vi "LVClass_WavefrontCorrector Reset to Factory WavefrontCorrectorSet.vi"(0 "WavefrontCorrector in":refnum<class "WavefrontCorrector.lvclass">, 5 "load_and_apply_connection_params":bool, 7 "load_and_apply_params":bool, 11 "error in (no error)":errorcluster) -> (4 "WavefrontCorrector out":refnum<class "WavefrontCorrector.lvclass">, 15 "error out":errorcluster)   [LabVIEW 2020, in "WavefrontCorrector.lvclass"]
doc: "Wavefront corrector parameter getter for parameter of type string.\n\n--------------------------------------------------------------------------------\n\n<B>correctorIn </B> : WavefrontCorrector object.\n<B>correctorOut </B> : WavefrontCorrector object.\n<B>parameter_name </B> : Name of the parameter.\n<B>value </B> : Value of the parameter.\n<B>ErrorIn </B> : Error\n<B>ErrorOut </B> : Error\n\n--------------------------------------------------------------------------------"
uses:
  WavefrontCorrector.lvclass
  WavefrontCorrector.lvclass/WavefrontCorrector.ctl
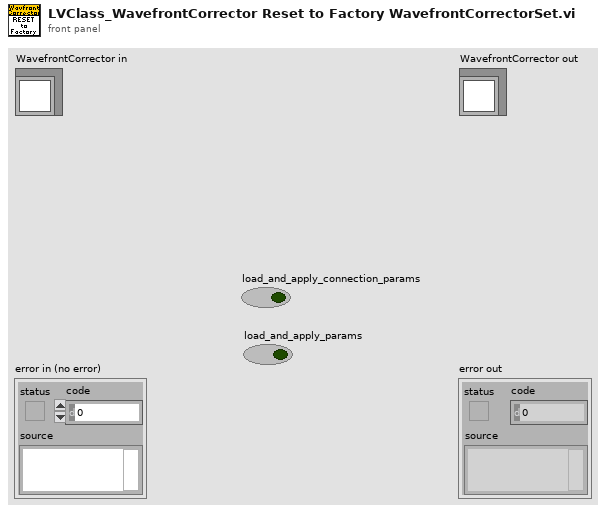
[diagram p1: front panel]
types:
  T1 = typedef "ClassID.ctl" = i64
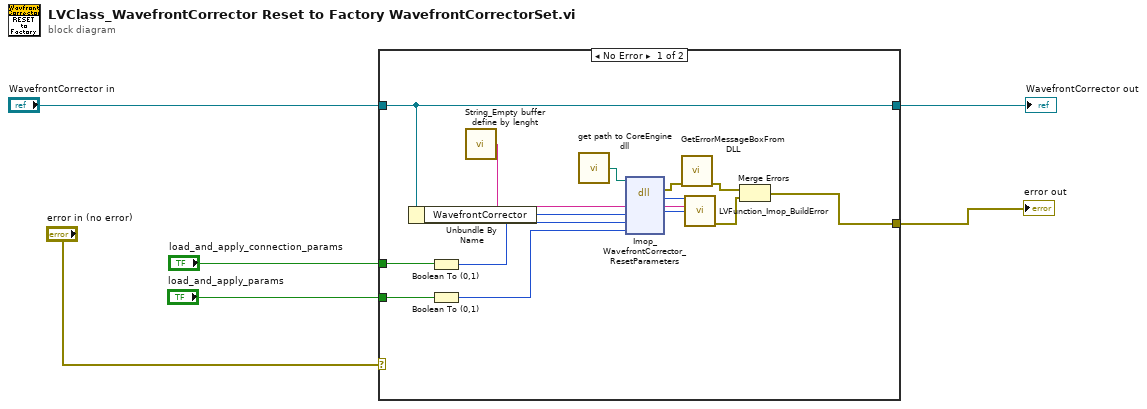
[diagram p0: block diagram]
diagram:
  n1 = case shown="No Error" "error in (no error)" {
    selector: "error in (no error)" -> [_ w23]
    tunnel: [w20 w23] -> w2
    tunnel: [w19 w22] -> w1
    tunnel: "WavefrontCorrector in" -> [w19 w22]
    tunnel: "load_and_apply_connection_params" -> [w11 _]
    tunnel: "load_and_apply_params" -> [w10 _]
    frame No Error {
      n2 = Unbundle By Name(w19) -> ("WavefrontCorrector"=w18:T1)
      n3 = Boolean To (0,1)(Boolean=w11) -> (0, 1=w8:i16)
      n4 = Boolean To (0,1)(Boolean=w10) -> (0, 1=w9:i16)
      n5 = call "String_Empty buffer define by lenght.vi"() -> ("Empty buffer"=w21:string)  [unwired: 1 in]
      n6 = call "get path to CoreEngine dll.vi"() -> ("path to wavekit library"=w15:path)  [unwired: 14 in, 1 out]
      n7 = dll-call lib="D:/soft/HASO_v3/SVN_trunk/ImOpCoreEngine4_LV2011/DLLs/c_interface_vc100.dll" fn="Imop_WavefrontCorrector_ResetParameters"(path in=w15, "message"=w21, "camera"=w18, "load_and_apply_connection_params"=w8, "load_and_apply_params"=w9) -> (error out=w14:errorcluster, "return type"=w16:i32, "message"=w17:string, "camera"=w7:i64)  [unwired: 4 in, 1 out]
      n8 = call "GetErrorMessageBoxFromDLL.vi"("error IN"=w14) -> ("error OUT"=w13:errorcluster)  [unwired: 10 in]
      n9 = call "LVFunction_Imop_BuildError.vi"("code"=w16, "String to Prepend to source (\"\")"=w17, "Adresse"=w7) -> ("error out"=w12:errorcluster)  [unwired: 12 in]
      n10 = Merge Errors(w13, w12) -> (w20:errorcluster)
    }
    frame Error {
    }
  }
  "error out" <- w2
  "WavefrontCorrector out" <- w1
